vi "Close.vi"(8 "error in (no error)":errorcluster, 11 "VISA resource name":refnum<visa-resource-name>) -> (0 "error out":errorcluster)   [LabVIEW 2020, in "Yokogawa GX Series.lvlib"]
doc: "Closes the I/O interface with the instrument."
uses:
  <instrlib>/Yokogawa GX Series/Yokogawa GX Series.lvlib
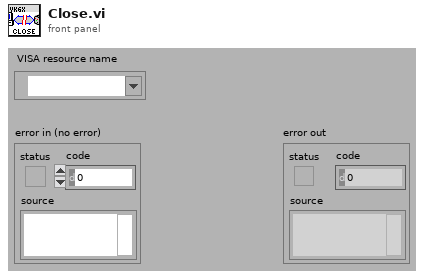
[diagram p1: front panel]
types:
  T1 = cluster{"User Name":string, "User ID":string, "Password":string, "Serial Auth Type (0: Not Auth)":u16, "SMARTDAC+ Type (0: Unknown)":u16, "Bluetooth Password":string}
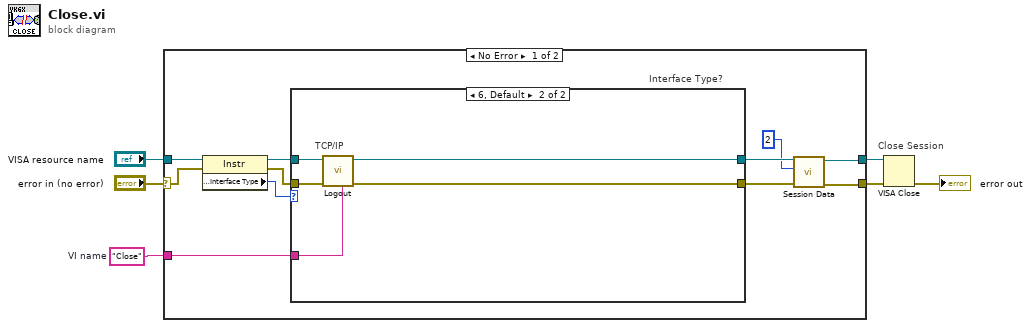
[diagram p0: block diagram]
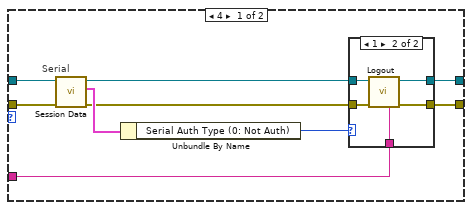
[diagram p2: hidden frame]
diagram:
  w5 = "Close"  # VI name
  # "Close Session"
  n1 = case shown="No Error" "error in (no error)" {
    selector: "error in (no error)" -> [w12 w39]
    tunnel: w5 -> [w17 _]
    tunnel: "VISA resource name" -> [w15 w40]
    tunnel: [w9 w40] -> w3
    tunnel: [w8 w39] -> w2
    frame No Error {
      n2 = property class="Instr"(reference=w15, error in=w12) -> (reference out=w14:refnum<visa-resource-name>, error out=w16:errorcluster, "Interface Information:Interface Type"=w13:u16)
      n3 = case "Interface Type?" shown="6, Default" w13 {
        tunnel: [w19 w38] -> w10
        tunnel: [w20 w37] -> w11
        tunnel: w17 -> [w21 w34]
        tunnel: w16 -> [w25 w35]
        tunnel: w14 -> [w26 w36]
        frame 4 {
          # "Serial"
          n4 = call <instrlib>:"Session Data.vi"("error in (no error)"=w25, "VISA resource name"=w26) -> ("error out"=w22:errorcluster, "User Data Out"=w24:T1, "VISA resource name out"=w23:refnum<visa-resource-name>)  [unwired: 7 in]
          n5 = Unbundle By Name(w24) -> ("Serial Auth Type (0: Not Auth)"=w18:u16)
          n6 = case shown="1" w18 {
            tunnel: w23 -> [w28 w33]
            tunnel: w22 -> [w27 w32]
            tunnel: [w28 w31] -> w20
            tunnel: [w27 w30] -> w19
            tunnel: w21 -> [_ w29]
            frame 0, Default {
            }
            frame 1 {
              n7 = call <instrlib>:"Logout.vi"("Source (\"\")"=w29, "error in (no error)"=w32, "VISA resource name"=w33) -> ("error out"=w30:errorcluster, "VISA resource name out"=w31:refnum<visa-resource-name>)  [unwired: 7 in]
            }
          }
        }
        frame 6, Default {
          # "TCP/IP"
          n8 = call <instrlib>:"Logout.vi"("Source (\"\")"=w34, "error in (no error)"=w35, "VISA resource name"=w36) -> ("error out"=w38:errorcluster, "VISA resource name out"=w37:refnum<visa-resource-name>)  [unwired: 7 out]
        }
      }
      n9 = call <instrlib>:"Session Data.vi"("error in (no error)"=w10, "Action (0 : Read Data)"=2, "VISA resource name"=w11) -> ("error out"=w8:errorcluster, "VISA resource name out"=w9:refnum<visa-resource-name>)  [unwired: 6 in, 1 out]
    }
    frame Error {
    }
  }
  n10 = VISA Close(VISA resource name=w3, error in (no error)=w2) -> (error out=→"error out":errorcluster)
